vi "Lvi Select Raw Format.vi"(8 "error in (no error)":errorcluster, 10 "RawFormat":bool, 11 "TaskRef":i32) -> (0 "error out":errorcluster, 2 "function return":i32, 3 "TaskRef out":i32)   [LabVIEW 2016, in "DtLvLink.lvlib"]
doc: "Calls directly into the entry points of the DLL of the Data Acq SDK to select whether the data from the task is in raw format or voltage. This VI is used by the higher-level VI, DtOLCreateTask."
uses:
  <userlib>/LV-Link3/DtLvLink.lvlib
  <userlib>/LV-Link3/DtLvLink_32.dll
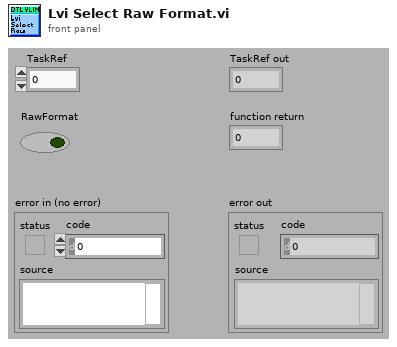
[diagram p1: front panel]
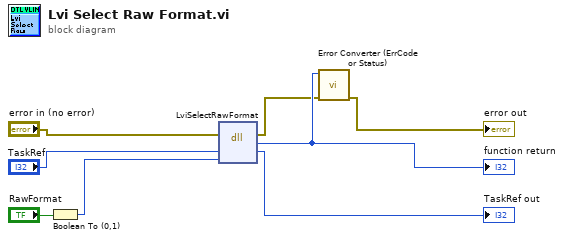
[diagram p0: block diagram]
diagram:
  n1 = Boolean To (0,1)(Boolean="RawFormat") -> (0, 1=w4:i16)
  n2 = dll-call lib="C:/Program Files (x86)/National Instruments/LabVIEW 2016/user.lib/LV-Link3/DtLvLink_32.*" fn="LviSelectRawFormat"(error in="error in (no error)", "TaskRef"="TaskRef", "RawFormat"=w4) -> (error out=w2:errorcluster, w8:i32, "TaskRef"=→"TaskRef out":i32)  [unwired: 3 in, 1 out]
  "function return" <- w8
  n3 = call <userlib>:"Error Converter (ErrCode or Status).vi"("error in (no error)"=w2, "error code"=w8) -> ("error out"=→"error out":errorcluster)  [unwired: 9 in]
